vi "CleanUp.vi"(0 "object in":refnum<class "Application.lvclass">, 5 "error in (no error)":errorcluster) -> (14 "object out":refnum<class "Application.lvclass">, 19 "error out":errorcluster)   [LabVIEW 2021, in "Application.lvclass"]
uses:
  Application.lvclass
  Application.lvclass/Application.ctl
  CetoniPump_class/CetoniPump.lvclass
  AD2_SDK_class/AD2_SDK.lvclass
  CoriFlowBFS1Plus_class/CoriFlowBFS1Plus.lvclass
  Hamamatsu_class/Hamamatsu.lvclass
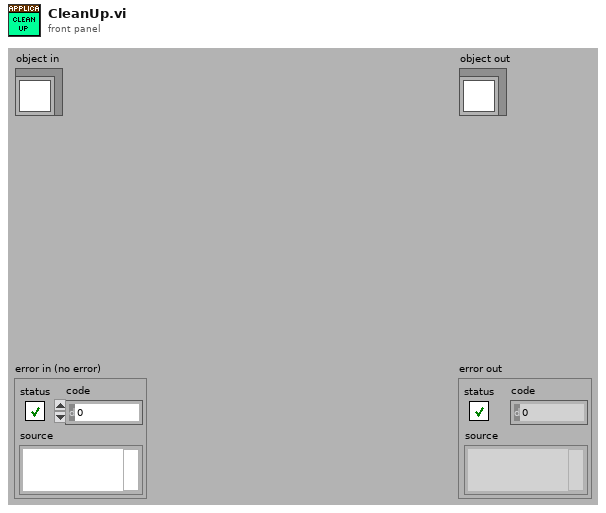
[diagram p1: front panel]
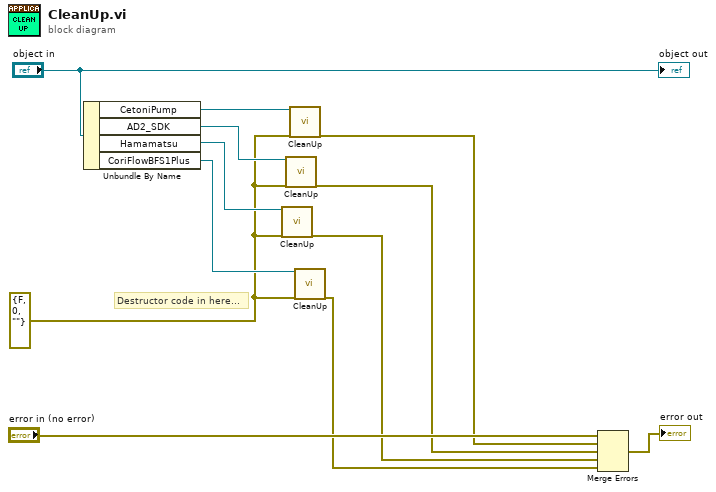
[diagram p0: block diagram]
diagram:
  w4 = errorcluster {"status"=FALSE, "code"=0, "source"=""} ("error in (no error)")
  # "Destructor code in here..."
  n1 = Unbundle By Name("object in") -> ("CetoniPump"=w9:refnum<class "CetoniPump.lvclass">, "AD2_SDK"=w7:refnum<class "AD2_SDK.lvclass">, "Hamamatsu"=w5:refnum<class "Hamamatsu.lvclass">, "CoriFlowBFS1Plus"=w6:refnum<class "CoriFlowBFS1Plus.lvclass">)
  n2 = call-dynamic "CleanUp.vi"("object in"=w5, "error in (no error)"=w4) -> ("error out"=w2:errorcluster)  [unwired: 16 in, 1 out]
  n3 = call-dynamic "CleanUp.vi"("object in"=w7, "error in (no error)"=w4) -> ("error out"=w3:errorcluster)  [unwired: 16 in, 1 out]
  n4 = call-dynamic "CleanUp.vi"("object in"=w9, "error in (no error)"=w4) -> ("error out"=w8:errorcluster)  [unwired: 16 in, 1 out]
  n5 = call-dynamic "CleanUp.vi"("object in"=w6, "error in (no error)"=w4) -> ("error out"=w1:errorcluster)  [unwired: 16 in, 1 out]
  n6 = Merge Errors("error in (no error)", w8, w3, w2, w1) -> (→"error out":errorcluster)
  "object out" <- "object in"
